vi "two data.vi"   [LabVIEW 2010]
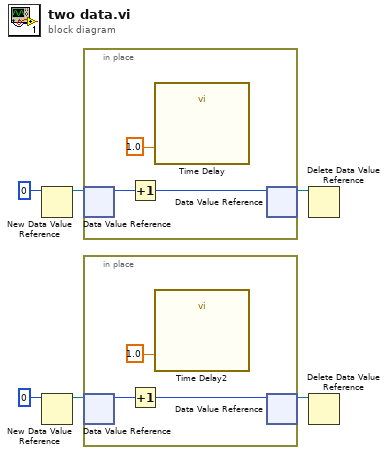
[diagram p0: block diagram]
diagram:
  n1 = New Data Value Reference(data value=0) -> (data value reference=w6:refnum<data-value>)  [unwired: 1 in, 1 out]
  n2 = New Data Value Reference(data value=0) -> (data value reference=w1:refnum<data-value>)  [unwired: 1 in, 1 out]
  n3 = in-place {
    n4 = in-place-dvr #1(w6) -> (w9:i32)  [unwired: 1 out]
    n5 = Increment(x=w9) -> (x+1=w8:i32)
    n6 = call "Time Delay"("Delay Time (s)"=1.0) -> ()  [unwired: 10 in, 1 out]
    n7 = in-place-dvr #1(w8) -> (w4:refnum<data-value>)  [unwired: 1 out]
  }
  n8 = in-place {
    n9 = in-place-dvr #2(w1) -> (w12:i32)  [unwired: 1 out]
    n10 = Increment(x=w12) -> (x+1=w11:i32)
    n11 = call "Time Delay2"("Delay Time (s)"=1.0) -> ()  [unwired: 10 in, 1 out]
    n12 = in-place-dvr #2(w11) -> (w3:refnum<data-value>)  [unwired: 1 out]
  }
  n13 = Delete Data Value Reference(data value reference=w4) -> ()  [unwired: 1 in, 2 out]
  n14 = Delete Data Value Reference(data value reference=w3) -> ()  [unwired: 1 in, 2 out]
